vi "MeasureCurrentonPowerSupply.vi"(10 "error in (no error)":errorcluster, 11 "VISA resource name":refnum<visa-resource-name>) -> (1 "Measurement":string, 2 "error out":errorcluster, 3 "VISA resource name out":refnum<visa-resource-name>)   [LabVIEW 2009]
uses:
  <instrlib>/BK Precision 91xx Series/BK Precision 91xx Series.lvlib
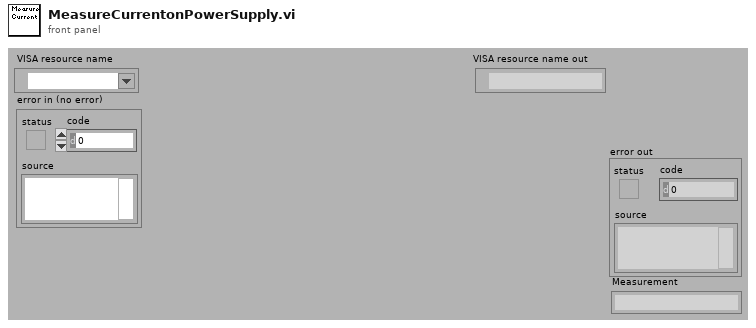
[diagram p1: front panel]
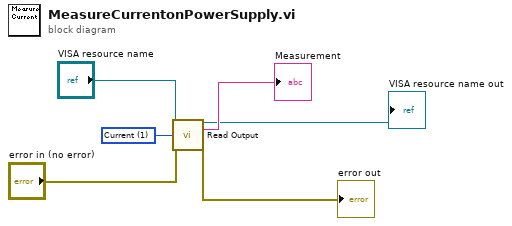
[diagram p0: block diagram]
diagram:
  w6 = u16 1 items=["Voltage", "Current", "Power", "Digital Volt Meter", "Resistance"] ("Measurement Function (0:Voltage)")
  n1 = call <instrlib>:"Read Output.vi"("VISA resource name"="VISA resource name", "Measurement Function (0:Voltage)"=w6, "error in (no error)"="error in (no error)") -> ("VISA resource name out"=→"VISA resource name out":refnum<visa-resource-name>, "Measurement"=→"Measurement":string, "error out"=→"error out":errorcluster)  [unwired: 10 in]
